vi "(x,y) to XY (single).vi"(8 "error in (no error)":errorcluster, 10 "[(x,y)]":cluster{"x":dbl, "y":dbl}[](array[cluster])) -> (0 "error out":errorcluster, 3 "XY-data out":cluster{"X-array":dbl[], "Y-array":dbl[]} {"Y-array" format="%.2p"; "X-array" format="%.2p"})   [LabVIEW 2019, in "xy_utilities.lvlib"]
doc: "Convert <b>XY-data</b> (cluster of arrays of X and Y) to <b>(x,y)</b> coordinates (array of clusters of (x,y) values).\n\nWire data to the data input to determine the polymorphic instance to use or manually select the instance."
uses:
  xy_utilities.lvlib
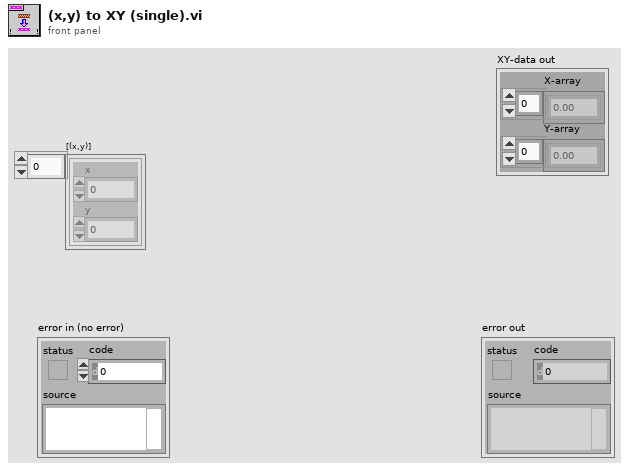
[diagram p1: front panel]
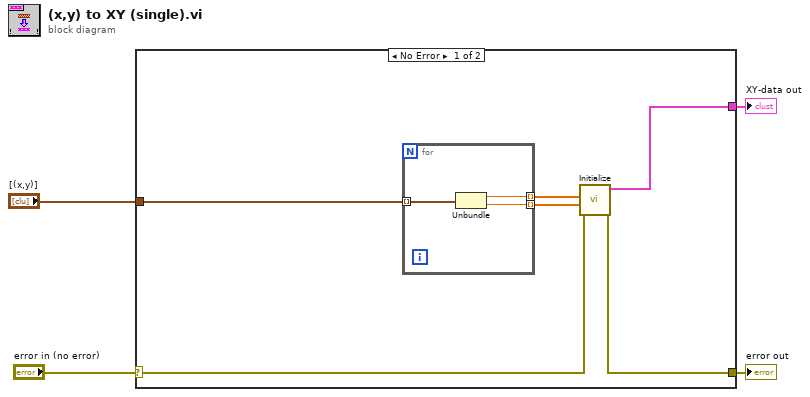
[diagram p0: block diagram]
diagram:
  n1 = case shown="No Error" "error in (no error)" {
    selector: "error in (no error)" -> [w7 w14]
    tunnel: [w6 w14] -> w3
    tunnel: [w5 _] -> w2
    tunnel: "[(x,y)]" -> [w10 _]
    frame No Error {
      n2 = for {
        tunnel: w10 -> [w13] mode=indexing
        tunnel: [w12] -> w9 mode=indexing
        tunnel: [w11] -> w8 mode=indexing
        n3 = Unbundle(w13) -> ("x"=w12:dbl, "y"=w11:dbl)
      }
      n4 = call "Initialize.vi"("error in (no error)"=w7, "Y-array"=w8, "X-array"=w9) -> ("error out"=w6:errorcluster, "XY-data out"=w5:cluster{"X-array":dbl[], "Y-array":dbl[]})  [unwired: 7 in]
    }
    frame Error {
    }
  }
  "error out" <- w3
  "XY-data out" <- w2
